vi "Core Actor - STOP - Internal Multithreading.vi"(8 "error in (no error)":errorcluster, 11 "Child_2_Class in":refnum<class "SW_Interface_Class.lvclass">) -> (0 "error out":errorcluster, 3 "Child_2_Class out":refnum<class "SW_Interface_Class.lvclass">)   [LabVIEW 2023, in "SW_Interface_Actor.lvlib" / "SW_Interface_Class.lvclass"]
uses:
  SW_Interface_Class.lvclass
  SW_Interface_Class.lvclass/SW_Interface_Class.ctl
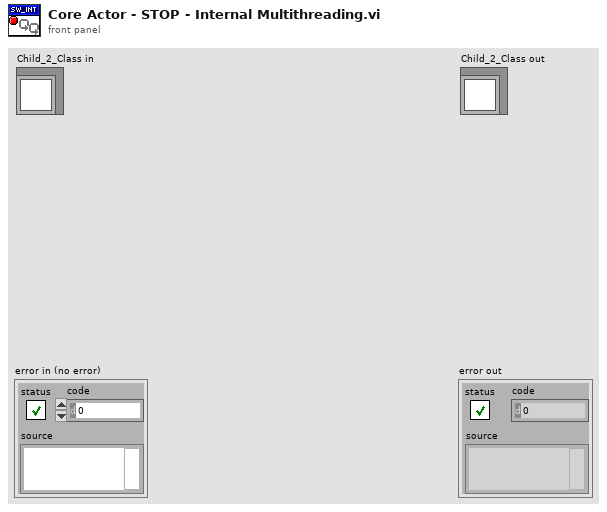
[diagram p1: front panel]
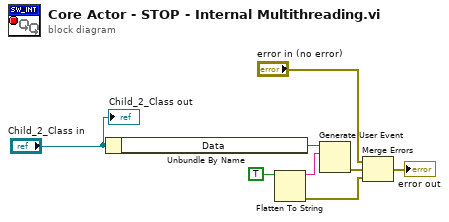
[diagram p0: block diagram]
diagram:
  n1 = Unbundle By Name("Child_2_Class in") -> ("Data"=w3:refnum<user-event>)
  n2 = Flatten To String(anything=TRUE) -> (data string=w7:string, error out=w4:errorcluster)  [unwired: 3 in, 1 out]
  n3 = Generate User Event(user event=w3, event data cluster=w7) -> (error out=w5:errorcluster)  [unwired: 2 in, 1 out]
  n4 = Merge Errors("error in (no error)", w5, w4) -> (→"error out":errorcluster)
  "Child_2_Class out" <- "Child_2_Class in"
